vi "Send Message.vi"(6 "priority":i32, 8 "error in (no error)":errorcluster, 9 "timeout ms (-1)":i32=-1, 10 "Message":refnum<class "Message.lvclass">, 11 "TCP Stream in":refnum<class "TCP Stream.lvclass">) -> (0 "error out":errorcluster, 3 "TCP Stream out":refnum<class "TCP Stream.lvclass">)   [LabVIEW 2020, in "TCP Stream.lvclass"]
uses:
  TCP Stream.lvclass
  G:/Utilisateurs/hugofroylan.aragon/Documents/PyCharm/neuro/labview/Nested Endpoint Actors/Abstract Classes/Message Stream/Message Stream.lvclass
  <vilib>/ActorFramework/Message/Message.lvclass
  Abstract Classes/Message Stream/Message Stream.lvclass/Message Stream.ctl
  TCP Stream.lvclass/TCP Stream.ctl
  Abstract Classes/Cipher/Cipher.lvclass
  Abstract Classes/Message Flattener/Message Flattener.lvclass
  Abstract Classes/Message Stream/Message Stream.lvclass
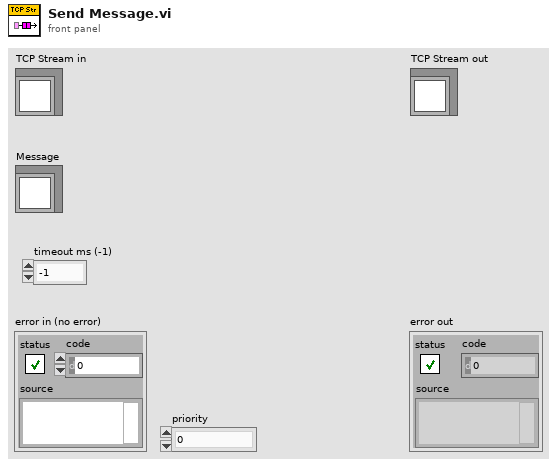
[diagram p1: front panel]
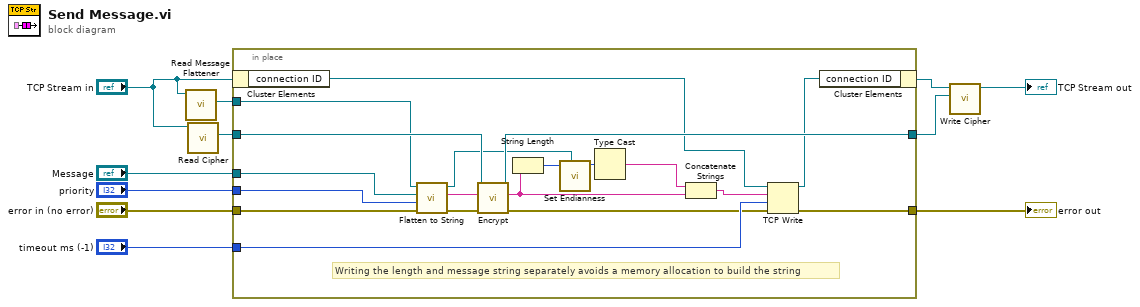
[diagram p0: block diagram]
diagram:
  n1 = call-dynamic "Read Message Flattener.vi"("Message Stream in"="TCP Stream in") -> ("Message Flattener.lvclass"=w1:refnum<class "Message Flattener.lvclass">)  [unwired: 9 in, 1 out]
  n2 = call "Read Cipher.vi"("Message Stream in"="TCP Stream in") -> ("Cipher.lvclass"=w5:refnum<class "Cipher.lvclass">)  [unwired: 10 in]
  n3 = in-place {
    in-place-border: "error in (no error)" -> [w24]
    in-place-border: w5 -> [w29]
    in-place-border: [w28] -> w3
    in-place-border: "priority" -> [w23]
    in-place-border: "Message" -> [w22]
    in-place-border: "timeout ms (-1)" -> [w19]
    in-place-border: [w26] -> w7
    in-place-border: w1 -> [w12]
    # "Writing the length and message string separately avoids a memory allocation to build the string"
    n4 = in-place-cluster #1("TCP Stream in") -> ("connection ID"=w18:refnum<k5>)
    n5 = call-dynamic "Flatten to String.vi"("error in (no error)"=w24, "priority"=w23, "Message"=w22, "Flattener in"=w12) -> ("error out"=w25:errorcluster, "Flattened String"=w21:string, "Flattener out"=w13:refnum<class "Message Flattener.lvclass">)  [unwired: 5 in]
    n6 = call-dynamic "Encrypt.vi"("error in (no error)"=w25, "Plaintext"=w21, "Cipher in"=w29) -> ("error out"=w14:errorcluster, "Cyphertext"=w16:string, "Cipher out"=w28:refnum<class "Cipher.lvclass">)  [unwired: 6 in]
    n7 = String Length(string=w16) -> (length=w30:i32)
    n8 = call-dynamic "Set Endianness.vi"("Message Flattener in"=w13, "bytes to read"=w30) -> ("bytes to read"=w20:i32)  [unwired: 9 in]
    n9 = Type Cast(x=w20) -> (*(type *) &x=w17:string)  [unwired: 1 in]
    n10 = Concatenate Strings(w17, w16) -> (w15:string)
    n11 = TCP Write(connection ID=w18, data in=w15, error in (no error)=w14, 9:w19) -> (connection ID out=w27:refnum<k5>, error out=w26:errorcluster)  [unwired: 1 out]
    n12 = in-place-cluster #1("connection ID"=w27) -> (w4:refnum<class "TCP Stream.lvclass">)
  }
  "error out" <- w7
  n13 = call "Write Cipher.vi"("Cipher"=w3, "Message Stream in"=w4) -> ("Message Stream out"=→"TCP Stream out":refnum<class "TCP Stream.lvclass">)  [unwired: 9 in]
